vi "Working with Nested Objects.vi"() -> ()   [LabVIEW 2015]
uses:
  <vilib>/NI/JSON Support for LabVIEW/JSON Data Classes/JSON Object/Insert Key Value Pair.vi
  <vilib>/NI/JSON Support for LabVIEW/JSON Data Classes/JSON Object/Insert Key Value Pair (Single String).vi
  <vilib>/NI/JSON Support for LabVIEW/JSON Data Classes/JSON Object/Insert Key Value Pair (Single Numeric).vi
  <vilib>/NI/JSON Support for LabVIEW/JSON Data Classes/JSON Object/Insert Key Value Pair (Single Boolean).vi
  <vilib>/NI/JSON Support for LabVIEW/JSON Data Classes/JSON Helper/New JSON.vi
  <vilib>/NI/JSON Support for LabVIEW/JSON Data Classes/JSON String/New JSON String.vi
  <vilib>/NI/JSON Support for LabVIEW/JSON Data Classes/JSON Array/New JSON Array (JSON Data).vi
  <vilib>/NI/JSON Support for LabVIEW/JSON Data Classes/JSON Object/Insert Key Value Pair (Single).vi
  <vilib>/NI/JSON Support for LabVIEW/JSON Data Classes/JSON Object/Get Value by Array (String Value).vi
  <vilib>/NI/JSON Support for LabVIEW/JSON Data Classes/JSON Object/Get Value by Array (Numeric Value).vi
  <vilib>/NI/JSON Support for LabVIEW/JSON Data Classes/JSON Object/Get Value by Array (Boolean Value).vi
  <vilib>/NI/JSON Support for LabVIEW/JSON Data Classes/JSON Object/Insert Key Value Pair (Nested String).vi
  <vilib>/NI/JSON Support for LabVIEW/JSON Data Classes/JSON Object/JSON Object.lvclass
  <vilib>/NI/JSON Support for LabVIEW/JSON Data Classes/JSON Object/Set Object Parameters XNode/Set Object Parameters.xnode
  <vilib>/NI/JSON Support for LabVIEW/JSON Data Classes/JSON Array/Build Array XNode/Build JSON Array.xnode
  <vilib>/NI/JSON Support for LabVIEW/JSON Data Classes/JSON Array/JSON Array.lvclass
  <vilib>/NI/JSON Support for LabVIEW/JSON Data Classes/JSON Datatype/JSON Null.lvclass
  <vilib>/NI/JSON Support for LabVIEW/JSON Data Classes/JSON Object/Get Parameter XNode/Get Object Parameters.xnode
  <vilib>/NI/JSON Support for LabVIEW/JSON Data Classes/JSON Helper/JSON Helper.lvclass
  <vilib>/NI/JSON Support for LabVIEW/JSON Data Classes/JSON String/JSON String.lvclass
panel:
  out "Modified Object":string
  out "array[1]":string
  out "array[0].key2":bool
  out "array[0].key1":dbl
  out "array[0].key0":string
  out "obj0.key2":bool
  out "obj0.key1":dbl
  out "obj0.key0":string
  out "Original Object":string
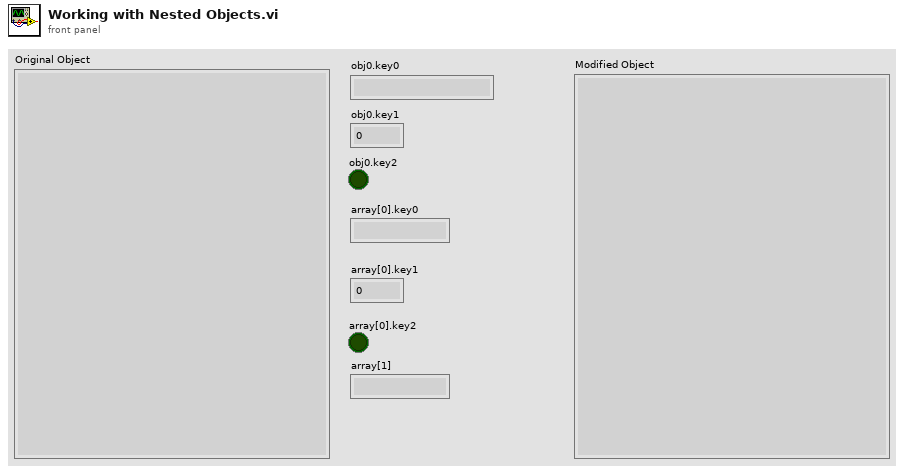
[diagram p1: front panel]
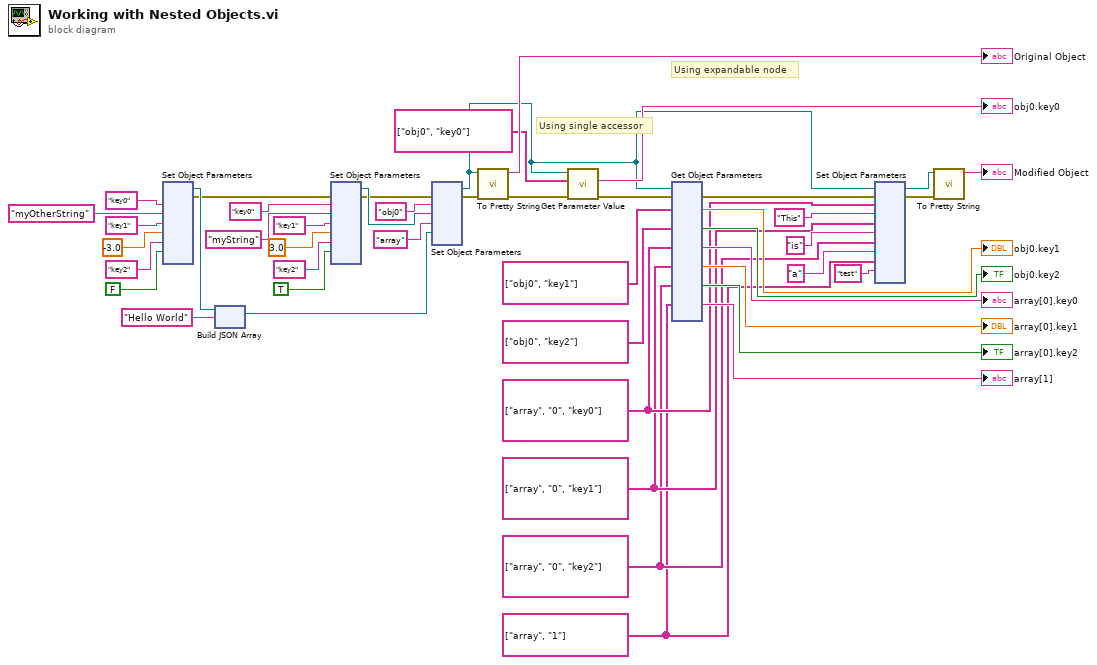
[diagram p0: block diagram]
diagram:
  w8 = string[] ["array", "1"] ("key")
  w9 = string[] ["array", "0", "key2"] ("key")
  w10 = string[] ["array", "0", "key1"] ("key")
  w11 = string[] ["array", "0", "key0"] ("key")
  # "Using expandable node"
  # "Using single accessor"
  n1 = xnode "Set Object Parameters"("key"="key0", "key"="key1", "key"="key2", "parameter"="myOtherString" ("key"), "parameter"=-3.0, "parameter"=FALSE) -> ("JSON Object Out"=w24:refnum<class "JSON Object.lvclass">, "error out"=w1:errorcluster)  [unwired: 2 in, 3 out]
  n2 = xnode "Build JSON Array"("input0"=w24, "input1"="Hello World" ("key")) -> ("JSON Array Out"=w23:refnum<class "JSON Array.lvclass">)
  n3 = xnode "Set Object Parameters"("key"="key0", "key"="key1", "key"="key2", "parameter"="myString" ("key"), "parameter"=3.0, "parameter"=TRUE, "error in"=w1) -> ("JSON Object Out"=w40:refnum<class "JSON Object.lvclass">, "error out"=w2:errorcluster)  [unwired: 1 in, 3 out]
  n4 = xnode "Set Object Parameters"("key"="obj0", "key"="array", "parameter"=w40, "parameter"=w23, "error in"=w2) -> ("JSON Object Out"=w20:refnum<class "JSON Object.lvclass">, "error out"=w3:errorcluster)  [unwired: 1 in, 2 out]
  n5 = call-dynamic "To Pretty String.vi"("error in (no error)"=w3, "JSON Object in"=w20) -> ("error out"=w7:errorcluster, "Pretty Print String"=→"Original Object":string)  [unwired: 8 in]
  n6 = call-poly <vilib>:"Get Parameter Value.vi"("error in (no error)"=w7, "Keys"=string[] ["obj0", "key0"] ("key"), "JSON Object in"=w20) -> ("error out"=w6:errorcluster, "value"=→"obj0.key0":string)  [unwired: 7 in]
  n7 = xnode "Get Object Parameters"("key"=string[] ["obj0", "key1"], "key"=string[] ["obj0", "key2"], "key"=w11, "key"=w10, "key"=w9, "key"=w8, "JSON Object In"=w20, "error in"=w6) -> ("parameter"=→"obj0.key1":dbl, "parameter"=→"obj0.key2":bool, "parameter"=→"array[0].key0":string, "parameter"=→"array[0].key1":dbl, "parameter"=→"array[0].key2":bool, "parameter"=→"array[1]":string, "error out"=w5:errorcluster)
  n8 = xnode "Set Object Parameters"("key"=w11, "key"=w10, "key"=w9, "key"=w8, "parameter"="This" ("key"), "parameter"="is" ("key"), "parameter"="a" ("key"), "parameter"="test" ("key"), "JSON Object In"=w20, "error in"=w5) -> ("JSON Object Out"=w13:refnum<class "JSON Object.lvclass">, "error out"=w4:errorcluster)  [unwired: 4 out]
  n9 = call-dynamic "To Pretty String.vi"("error in (no error)"=w4, "JSON Object in"=w13) -> ("Pretty Print String"=→"Modified Object":string)  [unwired: 8 in, 1 out]
